vi "LifeTimeImagePoint.vi"(0 "Boolean in":refnum<vi>, 3 "String":string, 4 "reference 6":refnum<vi>, 5 "String 2":string, 6 "reference 7":refnum<vi>, 7 "error in (no error)":errorcluster, 8 "reference 4":refnum<vi>, 10 "reference 3":refnum<vi>, 11 "reference 9":refnum<vi>, 12 "reference in":refnum<vi>, 13 "DigNum Refnum":refnum<vi>, 14 "Numeric in":i32, 15 "Str Refnum":refnum<vi>, 16 "X Stepsize":dbl, 18 "Array in":i32[][](array[numeric]), 19 "Point Measurement":refnum<vi>) -> (20 "Array out":i32[][](array[numeric]), 21 "CCD Chip Size":i32, 22 "X Start":dbl, 23 "Numeric out":dbl, 27 "error out":errorcluster)   [LabVIEW 2011]
uses:
  Program Files/Andor SOLIS/Drivers/Examples/LabVIEW/System Files/user.lib/atmcd32d.llb/Error Code Enum typedef.ctl
  Camera/vi/ccdChipPixels.vi
  Camera/vi/CamDef.vi
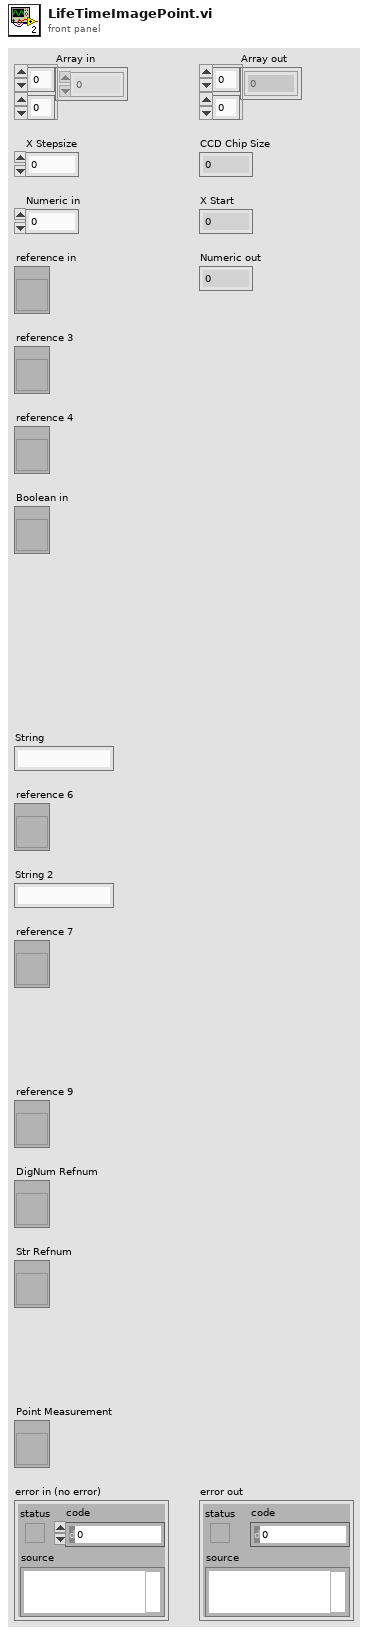
[diagram p1: front panel]
types:
  T1 = enum16{"No Measurement", "Aquire Image", "Point Measurement", "Multi Measurement", "Save Color Image"}
  T2 = enum16{"No Measurement", "Aquire Image", "Point Measurement", "Multi Measurement", "Save Color Image", "Find Single Mol.", "Auto Measurement Control", "Auto Point", "Aquire Line Scan", "Grid Measurement", "Trapping", "Move Scanner"}
  T3 = typedef "Error Code Enum typedef.ctl" = enum32{"N/A (0)", "DRV_ERROR_CODES", "DRV_SUCCESS", "DRV_VXDNOTINSTALLED", "DRV_ERROR_SCAN", "DRV_ERROR_CHECK_SUM", "DRV_ERROR_FILELOAD", "DRV_UNKNOWN_FUNC", "DRV_ERROR_VXD_INIT", "DRV_ERROR_ADDRESS", "DRV_ERROR_PAGELOCK", "DRV_ERROR_PAGEUNLOCK", "DRV_ERROR_BOARDTEST", "DRV_ERROR_ACK", "DRV_ERROR_UP_FIFO", "DRV_ERROR_PATTERN", "N/A (16)", "DRV_ACQUISITION_ERRORS", "DRV_ACQ_BUFFER", "DRV_ACQ_DOWNFIFO_FULL", "DRV_PROC_UNKONWN_INSTRUCTION", "DRV_ILLEGAL_OP_CODE", "DRV_KINETIC_TIME_NOT_MET", "DRV_ACCUM_TIME_NOT_MET", "DRV_NO_NEW_DATA", "N/A (25)", "DRV_SPOOLERROR", "N/A (27)", "N/A (28)", "N/A (29)", "N/A (30)", "N/A (31)", "N/A (32)", "DRV_TEMPERATURE_CODES", "DRV_TEMPERATURE_OFF", "DRV_TEMPERATURE_NOT_STABILIZED", "DRV_TEMPERATURE_STABILIZED", "DRV_TEMPERATURE_NOT_REACHED", "DRV_TEMPERATURE_OUT_RANGE", "DRV_TEMPERATURE_NOT_SUPPORTED", "DRV_TEMPERATURE_DRIFT", "N/A (41)", "N/A (42)", "N/A (43)", "N/A (44)", "N/A (45)", "N/A (46)", "N/A (47)", "N/A (48)", "DRV_GENERAL_ERRORS", "DRV_INVALID_AUX", "DRV_COF_NOTLOADED", "DRV_FPGAPROG", "DRV_FLEXERROR", "DRV_GPIBERROR", "N/A (55)", "N/A (56)", "N/A (57)", "N/A (58)", "N/A (59)", "N/A (60)", "N/A (61)", "N/A (62)", "N/A (63)", "DRV_DATATYPE", "DRV_DRIVER_ERRORS", "DRV_P1INVALID", "DRV_P2INVALID", "DRV_P3INVALID", "DRV_P4INVALID", "DRV_INIERROR", "DRV_COFERROR", "DRV_ACQUIRING", "DRV_IDLE", "DRV_TEMPCYCLE", "DRV_NOT_INITIALIZED", "DRV_P5INVALID", "DRV_P6INVALID", "DRV_INVALID_MODE", "DRV_INVALID_FILTER", "DRV_I2CERRORS", "DRV_I2CDEVNOTFOUND", "DRV_I2CTIMEOUT", "DRV_P7INVALID", "N/A (84)", "N/A (85)", "N/A (86)", "N/A (87)", "N/A (88)", "N/A (89)", "DRV_IOCERROR", "DRV_VRMVERSIONERROR"}
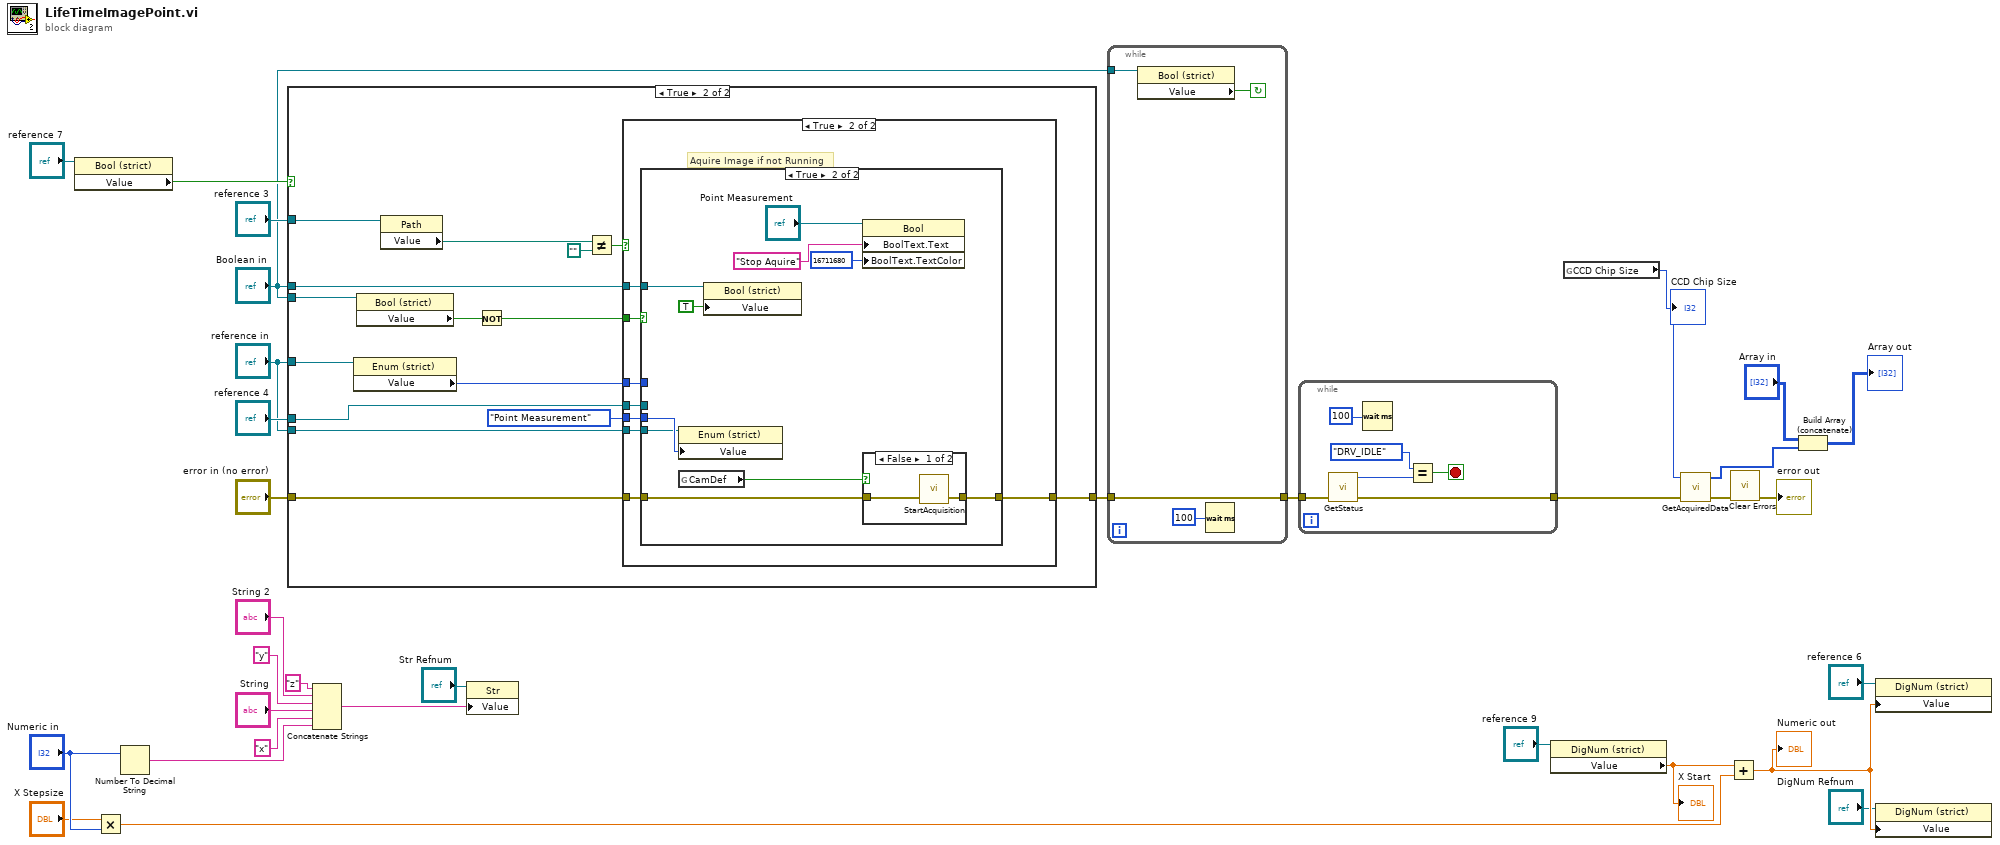
[diagram p0: block diagram]
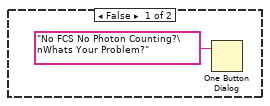
[diagram p2: hidden frame]
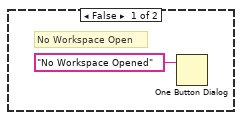
[diagram p3: hidden frame]
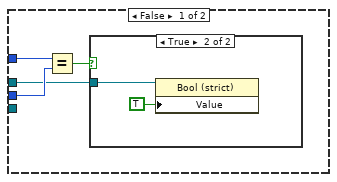
[diagram p4: hidden frame]
diagram:
  n1 = property class="Bool (strict)"(reference="reference 7") -> ("Value"=w20:bool)  [unwired: 1 in, 2 out]
  n2 = Multiply(x="X Stepsize", y="Numeric in") -> (x*y=w21:dbl)
  n3 = Number To Decimal String(number="Numeric in") -> (decimal integer string=w19:string)  [unwired: 1 in]
  n4 = case shown="True" w20 {
    tunnel: [_ w42] -> w11
    tunnel: "error in (no error)" -> [_ w41]
    tunnel: "Boolean in" -> [_ w39]
    tunnel: "reference in" -> [_ w38]
    tunnel: "reference 3" -> [_ w37]
    tunnel: "reference 4" -> [_ w36]
    tunnel: "reference in" -> [_ w35]
    tunnel: "Boolean in" -> [_ w34]
    frame False {
      n5 = One Button Dialog(message="No FCS No Photon Counting?\nWhats Your Problem?") -> ()  [unwired: 1 in, 1 out]
    }
    frame True {
      n6 = property class="Enum (strict)"(reference=w38) -> ("Value"=w47:T2)  [unwired: 1 in, 2 out]
      n7 = property class="Bool (strict)"(reference=w39) -> ("Value"=w48:bool)  [unwired: 1 in, 2 out]
      n8 = property class="Path"(reference=w37) -> ("Value"=w40:path)  [unwired: 1 in, 2 out]
      n9 = Not(x=w48) -> (.not. x?=w43:bool)
      n10 = Not Equal?(x=w40, y=path "") -> (x != y?=w44:bool)
      n11 = case shown="True" w44 {
        tunnel: w43 -> [_ w57]
        tunnel: T1."Point Measurement" ("Do Measurement") -> [_ w56]
        tunnel: w47 -> [_ w55]
        tunnel: [_ w54] -> w42
        tunnel: w41 -> [_ w53]
        tunnel: w36 -> [_ w52]
        tunnel: w35 -> [_ w51]
        tunnel: w34 -> [_ w50]
        frame False {
          # "No Workspace Open"
          n12 = One Button Dialog(message="No Workspace Opened") -> ()  [unwired: 1 in, 1 out]
        }
        frame True {
          # "Aquire Image if not Running"
          n13 = case shown="True" w57 {
            tunnel: w56 -> [w60 w71]
            tunnel: w55 -> [w61 _]
            tunnel: [_ w68] -> w54
            tunnel: w53 -> [_ w67]
            tunnel: w52 -> [w58 _]
            tunnel: w51 -> [_ w65]
            tunnel: w50 -> [_ w64]
            frame False {
              n14 = Equal?(x=w61, y=w60) -> (x = y?=w59:bool)
              n15 = case shown="True" w59 {
                tunnel: w58 -> [_ w62]
                frame False {
                }
                frame True {
                  n16 = property class="Bool (strict)"(reference=w62, "Value"=TRUE ("Stop Measurement")) -> ()  [unwired: 1 in, 2 out]
                }
              }
            }
            frame True {
              n17 = property class="Enum (strict)"(reference=w65, "Value"=w71) -> ()  [unwired: 1 in, 2 out]
              n18 = global read "CamDef.vi" "CamDef"() -> (w66:bool)
              n19 = property class="Bool (strict)"(reference=w64, "Value"=TRUE ("Measurement Running")) -> ()  [unwired: 1 in, 2 out]
              n20 = property on="Property Node" class="Bool"(reference="Point Measurement", "BoolText.Text"="Stop Aquire" ("Caption.Text"), "BoolText.TextColor"=u32 16711680 ("Boolean Text.Colors:FG Color")) -> ()  [unwired: 1 in, 2 out]
              n21 = case shown="False" w66 {
                tunnel: [w74 w76] -> w68
                tunnel: w67 -> [w75 w76]
                frame False {
                  n22 = call "StartAcquisition.vi"("error in (no error)"=w75) -> ("error out"=w74:errorcluster)  [unwired: 1 in, 1 out]
                }
                frame True {
                }
              }
            }
          }
        }
      }
    }
  }
  n23 = Concatenate Strings("z" ("string"), "String 2", "y" ("string"), "String", "x" ("string"), w19) -> (w32:string)
  n24 = property on="Property Node" class="Str"(reference="Str Refnum", "Value"=w32) -> ()  [unwired: 1 in, 2 out]
  n25 = while {
    tunnel: w11 -> [w77]
    tunnel: [w77] -> w24
    tunnel: "Boolean in" -> [w78]
    stop <- w80 continue-if-true
    n26 = property class="Bool (strict)"(reference=w78) -> ("Value"=w80:bool)  [unwired: 1 in, 2 out]
    n27 = Wait (ms)(milliseconds to wait=u32 100) -> ()  [unwired: 1 out]
  }
  n28 = while {
    tunnel: w24 -> [w81]
    tunnel: [w84] -> w23
    stop <- w83 stop-if-true
    n29 = call "GetStatus.vi"("error in (no error)"=w81) -> ("error out"=w84:errorcluster, "status"=w85:T3)  [unwired: 2 in, 1 out]
    n30 = Wait (ms)(milliseconds to wait=u32 100) -> ()  [unwired: 1 out]
    n31 = Equal?(x=Error_Code_Enum_typedef."DRV_IDLE" ("status"), y=w85) -> (x = y?=w83:bool)
  }
  n32 = property class="DigNum (strict)"(reference="reference 9") -> ("Value"=w29:dbl)  [unwired: 1 in, 2 out]
  "X Start" <- w29
  n33 = global read "ccdChipPixels.vi" "CCD Chip Size"() -> (w30:i32)
  "CCD Chip Size" <- w30
  n34 = call "GetAcquiredData.vi"("error in (no error)"=w23, "size"=w30) -> ("error out"=w25:errorcluster, "array"=w26:i32[])  [unwired: 1 in, 1 out]
  n35 = Add(x=w29, y=w21) -> (x+y=w31:dbl)
  "Numeric out" <- w31
  n36 = call <vilib>:"Clear Errors.vi"("error in (no error)"=w25) -> ("error out"=→"error out":errorcluster)  [unwired: 6 in]
  n37 = Build Array (concatenate)("Array in", w26) -> (→"Array out":i32[][])
  n38 = property class="DigNum (strict)"(reference="reference 6", "Value"=w31) -> ()  [unwired: 1 in, 2 out]
  n39 = property on="Property Node" class="DigNum (strict)"(reference="DigNum Refnum", "Value"=w31) -> ()  [unwired: 1 in, 2 out]
